vi "Release Notifier or Events.vi"(8 "error in (no error)":errorcluster, 11 "CallRequest (MsgPack) in":refnum<class "CallRequest (MsgPack).lvclass">) -> (0 "error out":errorcluster)   [LabVIEW 2020, in "wamplv.lvlib" / "CallRequest (MsgPack).lvclass"]
uses:
  CallRequest (MsgPack).lvclass
  CallRequest (MsgPack).lvclass/CallRequest (MsgPack).ctl
  c3bee624-ffbb-4308-a5ef-a601d606685f.vi
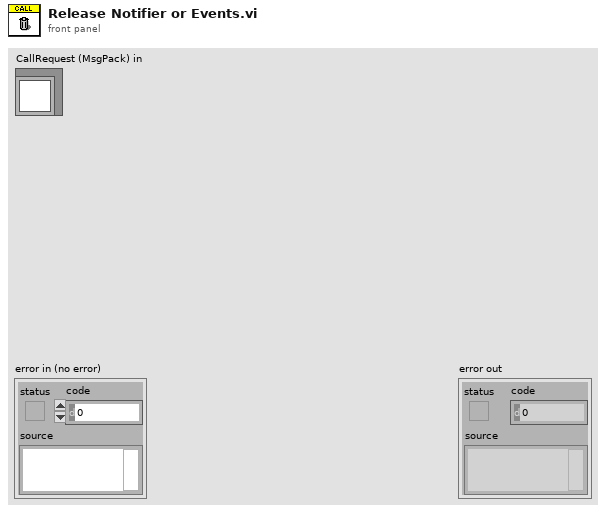
[diagram p1: front panel]
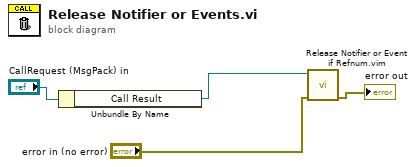
[diagram p0: block diagram]
diagram:
  n1 = Unbundle By Name("CallRequest (MsgPack) in") -> ("Call Result"=w3:refnum<notifier>)
  n2 = call "Release Notifier or Event if Refnum.vim"("error in (no error)"="error in (no error)", "Notifier or Event in"=w3) -> ("error out"=→"error out":errorcluster)  [unwired: 9 in]
